vi "tree issue.vi"() -> ()   [LabVIEW 2015]
panel:
  in  "stop":bool
  in  "length":i32
  in  "DS":T1(array[cluster])=[{"Left Cell String"="My Computer", "Child Text"=[""], "Child Tag"="My Computer", "Item Indent"=1, "Child Only?"=FALSE, "Glyph Index"=0}, {"Left Cell String"="Example1", "Child Text"=[""], "Child Tag"="My ComputerExample1", "Item Indent"=2, "Child Only?"=FALSE, "Glyph Index"=1}, {"Left Cell String"="Example2.vi", "Child Text"=["D:\\Soliton\\LabVIEW\\LV Project Viewer\\Example\\Example2.vi"], "Child Tag"="Example1Example2.vi", "Item Indent"=3, "Child Only?"=FALSE, "Glyph Index"=3}, {"Left Cell String"="Example4", "Child Text"=["D:\\Soliton\\LabVIEW\\LV Project Viewer\\Example\\Example4"], "Child Tag"="My ComputerExample4", "Item Indent"=2, "Child Only?"=FALSE, "Glyph Index"=1}, {"Left Cell String"="Example.lvclass", "Child Text"=["D:\\Soliton\\LabVIEW\\LV Project Viewer\\Example\\Example.lvclass"], "Child Tag"="My ComputerExample.lvclass", "Item Indent"=2, "Child Only?"=FALSE, "Glyph Index"=10}, {"Left Cell String"="Example.ctl", "Child Text"=["D:\\Soliton\\LabVIEW\\LV Project Viewer\\Example\\Example.lvclass\\Example.ctl"], "Child Tag"="Example.ctl", "Item Indent"=4, "Child Only?"=FALSE, "Glyph Index"=4}, {"Left Cell String"="Example3", "Child Text"=[""], "Child Tag"="Example3", "Item Indent"=4, "Child Only?"=FALSE, "Glyph Index"=1}, {"Left Cell String"="Example5.vi", "Child Text"=["D:\\Soliton\\LabVIEW\\LV Project Viewer\\Example\\Example5.vi"], "Child Tag"="Example3Example5.vi", "Item Indent"=5, "Child Only?"=FALSE, "Glyph Index"=3}, {"Left Cell String"="Example6.vi", "Child Text"=["D:\\Soliton\\LabVIEW\\LV Project Viewer\\Example\\Example6.vi"], "Child Tag"="Example3Example6.vi", "Item Indent"=5, "Child Only?"=FALSE, "Glyph Index"=3}, {"Left Cell String"="Numeric", "Child Text"=[""], "Child Tag"="Numeric", "Item Indent"=4, "Child Only?"=FALSE, "Glyph Index"=0}, {"Left Cell String"="Read Numeric.vi", "Child Text"=["D:\\Soliton\\LabVIEW\\LV Project Viewer\\Example\\Read Numeric.vi"], "Child Tag"="NumericRead Numeric.vi", "Item Indent"=5, "Child Only?"=FALSE, "Glyph Index"=3}, {"Left Cell String"="Write Numeric.vi", "Child Text"=["D:\\Soliton\\LabVIEW\\LV Project Viewer\\Example\\Write Numeric.vi"], "Child Tag"="NumericWrite Numeric.vi", "Item Indent"=5, "Child Only?"=FALSE, "Glyph Index"=3}, {"Left Cell String"="Example.lvlib", "Child Text"=["D:\\Soliton\\LabVIEW\\LV Project Viewer\\Example\\Example.lvlib"], "Child Tag"="My ComputerExample.lvlib", "Item Indent"=2, "Child Only?"=FALSE, "Glyph Index"=8}, {"Left Cell String"="Example2", "Child Text"=[""], "Child Tag"="Example2", "Item Indent"=4, "Child Only?"=FALSE, "Glyph Index"=1}, {"Left Cell String"="Example4.vi", "Child Text"=["D:\\Soliton\\LabVIEW\\LV Project Viewer\\Example\\Example4.vi"], "Child Tag"="Example2Example4.vi", "Item Indent"=5, "Child Only?"=FALSE, "Glyph Index"=3}, {"Left Cell String"="Example3.vi", "Child Text"=["D:\\Soliton\\LabVIEW\\LV Project Viewer\\Example\\Example3.vi"], "Child Tag"="Example3.vi", "Item Indent"=4, "Child Only?"=FALSE, "Glyph Index"=3}, {"Left Cell String"="Example1.ctl", "Child Text"=["D:\\Soliton\\LabVIEW\\LV Project Viewer\\Example\\Example1.ctl"], "Child Tag"="My ComputerExample1.ctl", "Item Indent"=2, "Child Only?"=FALSE, "Glyph Index"=4}, {"Left Cell String"="Example1.vi", "Child Text"=["D:\\Soliton\\LabVIEW\\LV Project Viewer\\Example\\Example1.vi"], "Child Tag"="My ComputerExample1.vi", "Item Indent"=2, "Child Only?"=FALSE, "Glyph Index"=3}, {"Left Cell String"="Dependencies", "Child Text"=[""], "Child Tag"="My ComputerDependencies", "Item Indent"=2, "Child Only?"=FALSE, "Glyph Index"=0}, {"Left Cell String"="vi.lib", "Child Text"=[""], "Child Tag"="Dependenciesvi.lib", "Item Indent"=3, "Child Only?"=FALSE, "Glyph Index"=1}, {"Left Cell String"="Clear Errors.vi", "Child Text"=[""], "Child Tag"="vi.libClear Errors.vi", "Item Indent"=4, "Child Only?"=FALSE, "Glyph Index"=3}, {"Left Cell String"="Build Specifications", "Child Text"=[""], "Child Tag"="My ComputerBuild Specifications", "Item Indent"=2, "Child Only?"=FALSE, "Glyph Index"=0}, {"Left Cell String"="My Application", "Child Text"=[""], "Child Tag"="Build SpecificationsMy Application", "Item Indent"=3, "Child Only?"=FALSE, "Glyph Index"=0}]
  in  "Tree":string(tree)
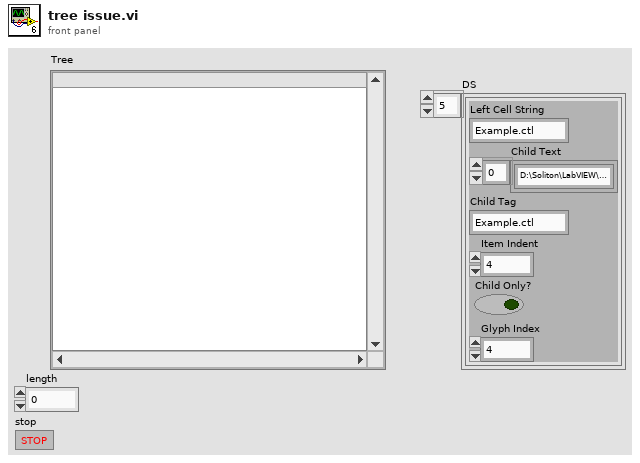
[diagram p1: front panel]
types:
  T1 = cluster{"Left Cell String":string, "Child Text":string[], "Child Tag":string, "Item Indent":i32, "Child Only?":bool, "Glyph Index":i32}[]
  T2 = cluster{"Left Cell String":string, "Child Text":string[], "Child Tag":string, "Item Indent":i32, "Child Only?":bool, "Glyph Index":i32}
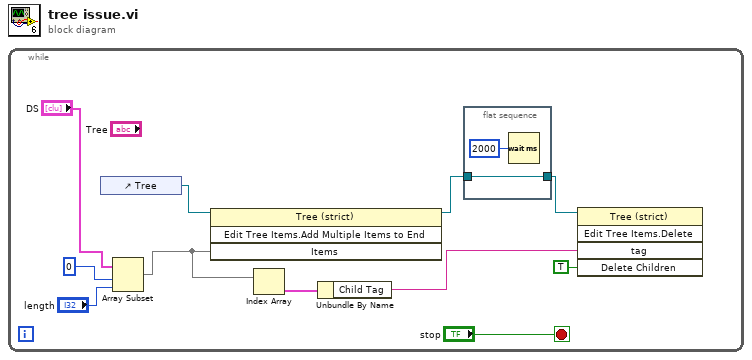
[diagram p0: block diagram]
diagram:
  n1 = while {
    stop <- "stop" stop-if-true
    n2 = control-ref of="Tree"() -> (w11:refnum<vi>)
    n3 = Array Subset(array="DS", index=0, length="length") -> (w4:T1)
    n4 = invoke class="Tree (strict)" method="Edit Tree Items.Add Multiple Items to End"(reference=w11, "Items"=w4) -> (reference out=w2:refnum<vi>)  [unwired: 2 in, 3 out]
    n5 = Index Array(array=w4) -> (element=w5:T2)  [unwired: 1 in]
    n6 = Unbundle By Name(w5) -> ("Child Tag"=w3:string)
    n7 = flat-sequence {
      tunnel: w2 -> [w12]
      tunnel: [w12] -> w1
      frame #0 {
        n8 = Wait (ms)(milliseconds to wait=u32 2000) -> ()  [unwired: 1 out]
      }
    }
    n9 = invoke class="Tree (strict)" method="Edit Tree Items.Delete"(reference=w1, "tag"=w3, "Delete Children"=TRUE ("Delete Children?")) -> ()  [unwired: 2 in, 5 out]
  }
